vi "Build Rotation Set.vi"(6 "Rotation Reduction":dbl=1.0, 7 "Rotate(Yaw) CCW 1 CW -1":dbl, 11 "Frame Set":T1 {"Back Right"."Angle" scale format="%.3f"; "Back Right"."Velocity" scale=-1.0..1.0 scale format="%.1f"; "Back Left"."Angle" scale format="%.3f"; "Back Left"."Velocity" scale=-1.0..1.0 scale format="%.1f"; "Front Left"."Angle" scale format="%.3f"; "Front Left"."Velocity" scale=-1.0..1.0 scale format="%.1f"; "Front Right"."Angle" scale format="%.3f"; "Front Right"."Velocity" scale=-1.0..1.0 scale format="%.1f"}) -> (3 "Rotation Set Out":T1 {"Back Right"."Angle" scale format="%.3f"; "Back Right"."Velocity" scale=-1.0..1.0 scale format="%.1f"; "Back Left"."Angle" scale format="%.3f"; "Back Left"."Velocity" scale=-1.0..1.0 scale format="%.1f"; "Front Left"."Angle" scale format="%.3f"; "Front Left"."Velocity" scale=-1.0..1.0 scale format="%.1f"; "Front Right"."Angle" scale format="%.3f"; "Front Right"."Velocity" scale=-1.0..1.0 scale format="%.1f"})   [LabVIEW 2020, in "SwerveDrive_ACT.lvlib"]
uses:
  SwerveDrive_ACT.lvlib
  Shared Code/TypeDefs/Cluster_Swerve 4 Steer and Velocity.ctl
  Shared Code/TypeDefs/Cluster_Module Velocity-Direction-Rotations.ctl
  Shared Code/TypeDefs/Level_Velocity plus-minus 1.ctl
  Shared Code/TypeDefs/Dial_Compase heading unit circle CCW positive.ctl
panel:
  # "\"Front\" of Robot"
  # "Right Hand Rule"
  # "X"
  # "+CCW"
  # "Y"
  # "(0,0)"
  # "\"Front\" of Robot"
  # "Right Hand Rule"
  # "X"
  # "+CCW"
  # "Y"
  # "(0,0)"
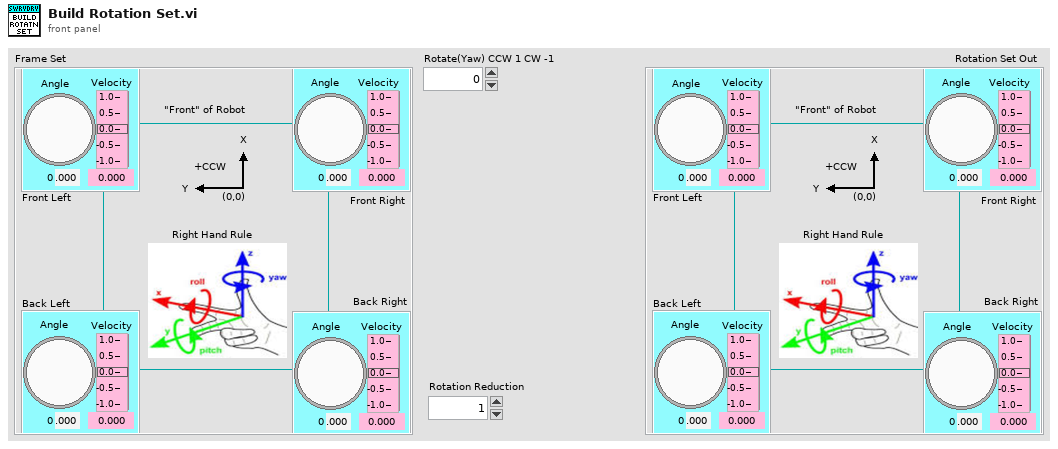
[diagram p1: front panel]
types:
  T1 = typedef "Cluster_Swerve 4 Steer and Velocity.ctl" = cluster{"Front Right":T2, "Front Left":T2, "Back Left":T2, "Back Right":T2}
  T2 = typedef "Cluster_Module Velocity-Direction-Rotations.ctl" = cluster{"Velocity":T3, "Angle":T4, "Rotations Count":dbl}
  T3 = typedef "Level_Velocity plus-minus 1.ctl" = dbl
  T4 = typedef "Dial_Compase heading unit circle CCW positive.ctl" = dbl
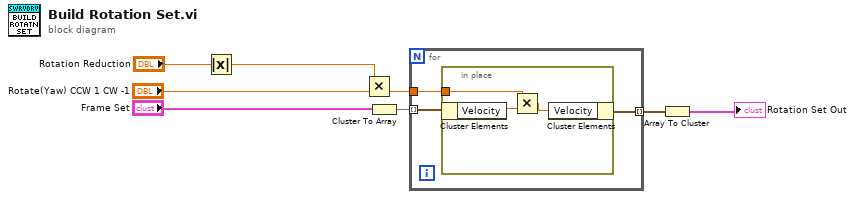
[diagram p0: block diagram]
diagram:
  n1 = Absolute Value(x="Rotation Reduction") -> (abs(x)=w1:dbl)
  n2 = Multiply(x=w1, y="Rotate(Yaw) CCW 1 CW -1") -> (x*y=w3:dbl)
  n3 = Cluster To Array(cluster="Frame Set") -> (array=w7:T2[])
  n4 = for {
    tunnel: w7 -> [w11] mode=indexing
    tunnel: w3 -> [w10]
    tunnel: [w9] -> w5 mode=indexing
    n5 = in-place {
      in-place-border: w10 -> [w12]
      n6 = in-place-cluster #1(w11) -> ("Velocity"=w14:T3)
      n7 = Multiply(x=w12, y=w14) -> (x*y=w13:T3)
      n8 = in-place-cluster #1("Velocity"=w13) -> (w9:T2)
    }
  }
  n9 = Array To Cluster(array=w5) -> (cluster=→"Rotation Set Out":cluster{"[0]":T2, "[1]":T2, "[2]":T2, "[3]":T2})
